vi "Start Message.vi"(10 "Index":u64, 11 "Message Number":u8) -> (2 "Position":u8, 3 "Message":u64)   [LabVIEW 2016, in "DCM-Classes.lvlib" / "DCM - RT - Tools.lvlib"]
uses:
  DCM - RT - Tools.lvlib
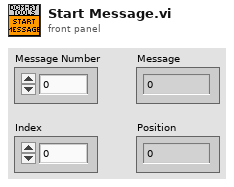
[diagram p1: front panel]
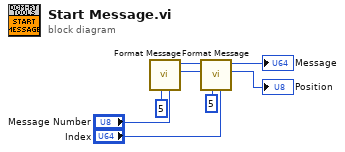
[diagram p0: block diagram]
diagram:
  n1 = call "Format Message.vi"("Value"="Message Number", "Size"=u8 5) -> ("Position"=w7:u8, "Message"=w6:u64)  [unwired: 8 in]
  n2 = call "Format Message.vi"("Value"="Index", "Size"=u8 5, "Position (0)"=w7, "Message"=w6) -> ("Position"=→"Position":u8, "Message"=→"Message":u64)  [unwired: 6 in]
